vi "save_dim2_array.vi"(8 "error in (no error)":errorcluster, 10 "2dim data array":string[][](array[string]), 11 "DataLogging in":refnum<class "DataLogging.lvclass">) -> (0 "error out":errorcluster, 3 "DataLogging out":refnum<class "DataLogging.lvclass">)   [LabVIEW 2017, in "DataLogging.lvclass"]
doc: "The input array (dim2) is being saved into the datafile/database.\nThe datalog object stores the path of the logfile and other\nparameters for each analysis"
uses:
  DataLogging.lvclass
  ValueArray.ctl
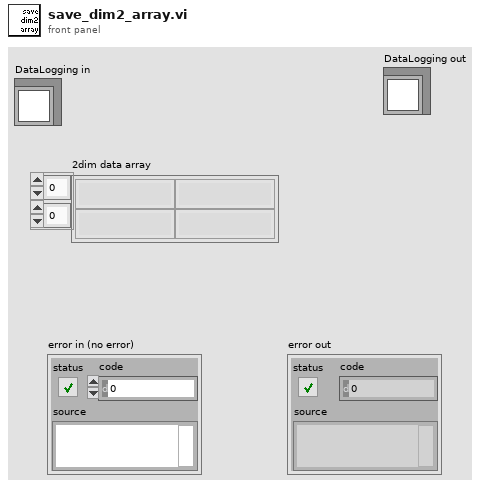
[diagram p1: front panel]
types:
  T1 = typedef "ValueArray.ctl" = string[]
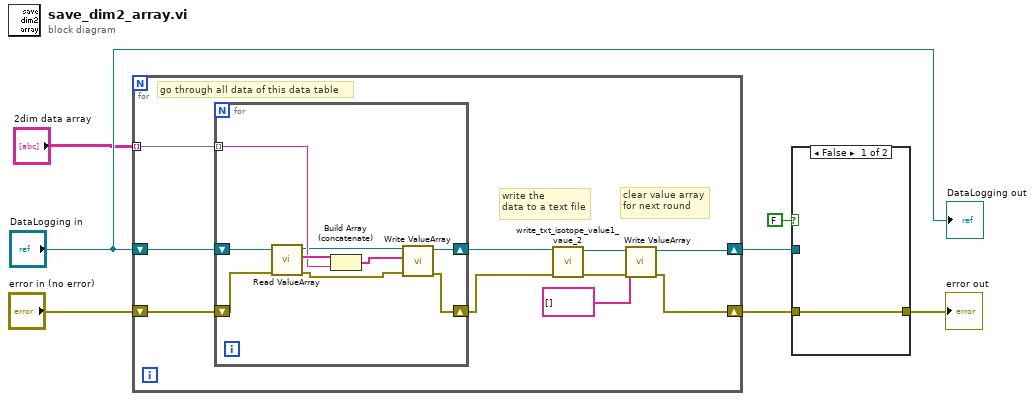
[diagram p0: block diagram]
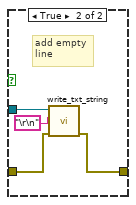
[diagram p2: hidden frame]
diagram:
  n1 = for {
    tunnel: "2dim data array" -> [w17] mode=indexing
    shift-right: [w9] -> w3
    shift-left: "error in (no error)" -> [w15]
    shift-right: [w10] -> w4
    shift-left: "DataLogging in" -> [w16]
    # "clear value array\nfor next round"
    # "write the\ndata to a text file"
    # "go through all data of this data table"
    n2 = for {
      tunnel: w17 -> [w23] mode=indexing
      shift-right: [w19] -> w14
      shift-left: w16 -> [w26]
      shift-right: [w18] -> w13
      shift-left: w15 -> [w25]
      n3 = call-dynamic "Read ValueArray.vi"("error in (no error)"=w25, "DataLogging in"=w26) -> ("error out"=w20:errorcluster, "ValueArray"=w24:T1, "DataLogging out"=w21:refnum<class "DataLogging.lvclass">)  [unwired: 7 in]
      n4 = Build Array (concatenate)(w24, w23) -> (w22:T1)
      n5 = call-dynamic "Write ValueArray.vi"("error in (no error)"=w20, "ValueArray"=w22, "DataLogging in"=w21) -> ("error out"=w18:errorcluster, "DataLogging out"=w19:refnum<class "DataLogging.lvclass">)  [unwired: 7 in]
    }
    n6 = call-dynamic "write_txt_isotope_value1_vaue_2.vi"("error in (no error)"=w13, "DataLoggingText in"=w14) -> ("error out"=w11:errorcluster, "DataLoggingText out"=w12:refnum<class "DataLogging.lvclass">)  [unwired: 8 in]
    n7 = call-dynamic "Write ValueArray.vi"("error in (no error)"=w11, "ValueArray"=T1 [], "DataLogging in"=w12) -> ("error out"=w9:errorcluster, "DataLogging out"=w10:refnum<class "DataLogging.lvclass">)  [unwired: 7 in]
  }
  n8 = case shown="False" FALSE {
    tunnel: w4 -> [_ w31]
    tunnel: w3 -> [w27 w29]
    tunnel: [w27 w28] -> w2
    frame False {
    }
    frame True {
      # "add empty\nline"
      n9 = call-dynamic "write_txt_string.vi"("error in (no error)"=w29, "data string"="\r\n", "DataLoggingText in"=w31) -> ("error out"=w28:errorcluster)  [unwired: 7 in, 1 out]
    }
  }
  "error out" <- w2
  "DataLogging out" <- "DataLogging in"
